vi "Shut_Down_EnFlo_Lab.vi"(0 "Initial Shutdown":bool) -> ()   [LabVIEW 2022 SP3]
uses:
  ADAM Client/Sub VIs/ADAM Controls/Function_ADAM.ctl
  ADAM Client/Sub VIs/ADAM Controls/Channel_State.ctl
  Channel_Description_Global.vi
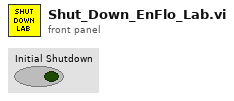
[diagram p1: front panel]
types:
  T1 = typedef "Ch_description_ADAM.ctl" = cluster{"Ch Name":string, "Type":T2, "Function":T3, "Ch State":T4, "Calibration type":T5, "A":dbl, "B":dbl, "C":dbl, "D":dbl, "Comments":string, "Address":T6, "String":string, "Duty":u16}
  T2 = typedef "Module_type_ADAM.ctl" = string
  T3 = typedef "Function_ADAM.ctl" = enum16{"Analogue Input", "Digital Input", "Event counter", "Event rate", "Analogue Output", "Digital Output", "Relay Output"}
  T4 = typedef "Channel_State.ctl" = enum16{"On", "Off", "Always On", "Always Off"}
  T5 = typedef "Calib_type_ADAM.ctl" = string
  T6 = typedef "Address.ctl" = cluster{"Main":i32, "Ch.":i32, "Sub":i32, "Port Name":string}
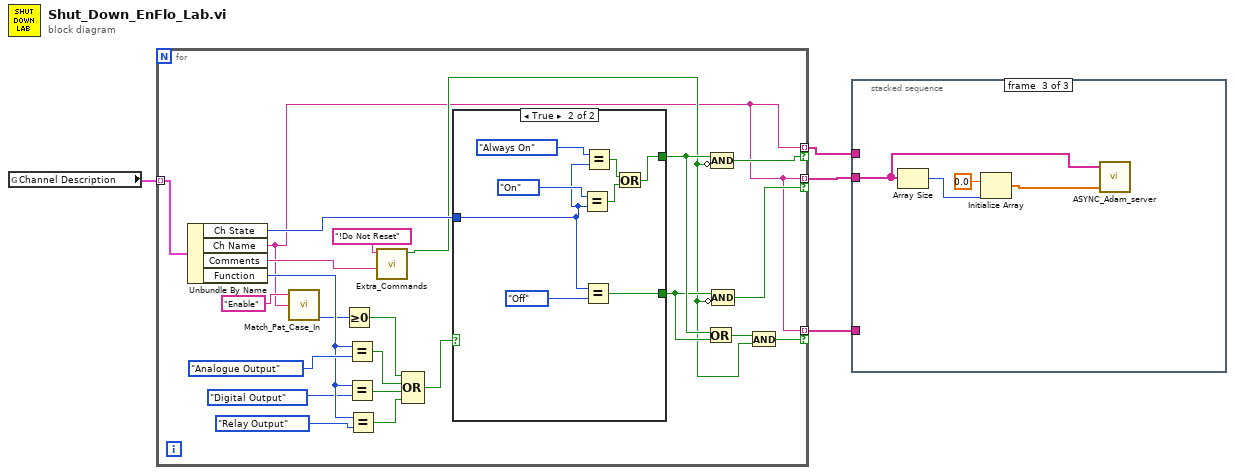
[diagram p0: block diagram]
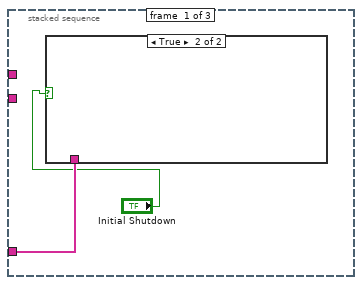
[diagram p2: hidden frame]
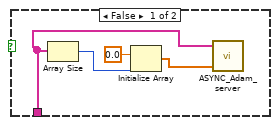
[diagram p3: hidden frame]
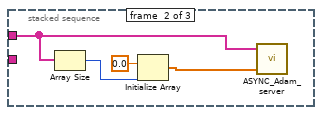
[diagram p4: hidden frame]
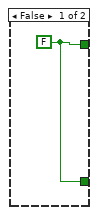
[diagram p5: hidden frame]
diagram:
  n1 = global read "Channel_Description_Global.vi" "Channel Description"() -> (w1:T1[])
  n2 = for {
    tunnel: w1 -> [w27] mode=indexing
    tunnel: [w7] -> w4 mode=indexing if=w15
    tunnel: [w7] -> w3 mode=indexing if=w14
    tunnel: [w7] -> w2 mode=indexing if=w9
    n3 = Unbundle By Name(w27) -> ("Ch State"=w17:T4, "Ch Name"=w7:string, "Comments"=w18:string, "Function"=w25:T3)
    n4 = call "Match_Pat_Case_In.vi"("String to match"="Enable" ("regular expression"), "String"=w7) -> ("offset past match"=w6:i32)  [unwired: 1 in, 3 out]
    n5 = Greater Or Equal To 0?(x=w6) -> (x >= 0?=w5:bool)
    n6 = Equal?(x=w25, y=Function_ADAM."Analogue Output" ("Function")) -> (x = y?=w22:bool)
    n7 = Equal?(x=w25, y=Function_ADAM."Digital Output" ("Function")) -> (x = y?=w21:bool)
    n8 = Equal?(x=w25, y=Function_ADAM."Relay Output" ("Function")) -> (x = y?=w20:bool)
    n9 = call "Extra_Commands.vi"("String to Search"=w18, "Command"="!Do Not Reset" ("String to match")) -> ("Command Found"=w10:bool)  [unwired: 1 in, 4 out]
    n10 = Compound Arithmetic op=OR(w5, w22, w21, w20) -> (w16:bool)
    n11 = case shown="True" w16 {
      tunnel: w17 -> [_ w31]
      tunnel: [w28 w30] -> w13
      tunnel: [w28 w29] -> w12
      frame False {
        w28 = FALSE
      }
      frame True {
        n12 = Equal?(x=Channel_State."On" ("Ch State"), y=w31) -> (x = y?=w33:bool)
        n13 = Equal?(x=w31, y=Channel_State."Off" ("Ch State")) -> (x = y?=w29:bool)
        n14 = Equal?(x=Channel_State."Always On" ("Ch State"), y=w31) -> (x = y?=w34:bool)
        n15 = Or(x=w34, y=w33) -> (x .or. y?=w30:bool)
      }
    }
    n16 = Or(x=w13, y=w12) -> (x .or. y?=w11:bool)
    n17 = Compound Arithmetic op=AND(w13, invert w10) -> (w15:bool)
    n18 = Compound Arithmetic op=AND(w12, invert w10) -> (w14:bool)
    n19 = And(x=w11, y=w10) -> (x .and. y?=w9:bool)
  }
  n20 = stacked-sequence {
    tunnel: w4 -> [_ w43 _]
    tunnel: w3 -> [_ _ w47]
    tunnel: w2 -> [w38 _ _]
    frame #0 {
      n21 = case shown="True" "Initial Shutdown" {
        tunnel: w38 -> [w39 _]
        frame False {
          n22 = Array Size(array=w39) -> (size(s)=w41:i32)
          n23 = Initialize Array(0.0 ("element"), w41) -> (w40:dbl[])
          n24 = call "ASYNC_Adam_server.vi"("Values"=w40, "Channel Names"=w39) -> ()  [unwired: 1 in, 3 out]
        }
        frame True {
        }
      }
    }
    frame #1 {
      n25 = Array Size(array=w43) -> (size(s)=w45:i32)
      n26 = Initialize Array(0.0 ("element"), w45) -> (w44:dbl[])
      n27 = call "ASYNC_Adam_server.vi"("Values"=w44, "Channel Names"=w43) -> ()  [unwired: 1 in, 3 out]
    }
    frame #2 {
      n28 = Array Size(array=w47) -> (size(s)=w49:i32)
      n29 = Initialize Array(0.0 ("element"), w49) -> (w48:dbl[])
      n30 = call "ASYNC_Adam_server.vi"("Values"=w48, "Channel Names"=w47) -> ()  [unwired: 1 in, 3 out]
    }
  }
